vi "getExptComments.vi"(8 "error in (no error)":errorcluster, 11 "Inst.Transport in":refnum<class "Inst.Transport.lvclass">) -> (0 "error out":errorcluster, 2 "comments":string, 3 "Inst.Transport out":refnum<class "Inst.Transport.lvclass">)   [LabVIEW 2019, in "Inst.Transport.lvclass"]
uses:
  Inst.Transport.lvclass
  Typedefs/Inst.Transport.PublicCommands--Enum.ctl
  Typedefs/ExptComments--RequestResponse--Cluster.ctl
  6c876aff-ff84-4813-ac9a-c50593048c18.vi
  6c876aff-ff84-4813-ac9a-c50593048c18.vi/f3aab538-2ba4-4839-a97a-c1727853db43.vi
  6c876aff-ff84-4813-ac9a-c50593048c18.vi/9b28f1f0-4a86-40ce-ac33-3c033e206612.vi
  <vilib>/Utility/Data Type/Get Type Information.vi
  <vilib>/JDP Science/JSONtext/JSON text to Variant.vi
  <vilib>/JDP Science/JSONtext/LVClass Serializer/JSONtext LVClass Serializer.lvclass
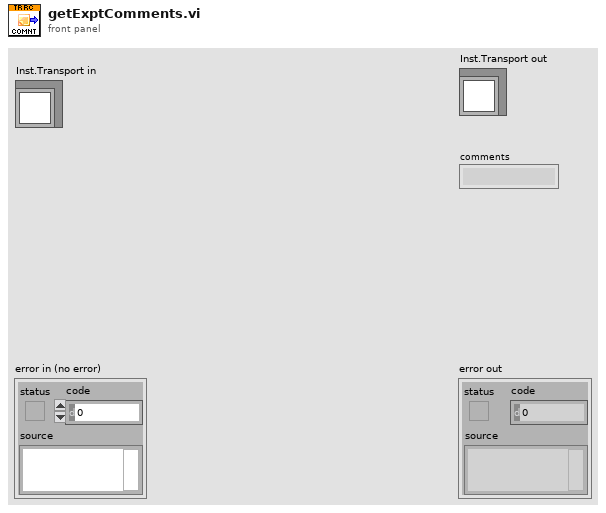
[diagram p1: front panel]
types:
  T1 = typedef "Inst.Transport.lvclass/ExptComments--RequestResponse--Cluster.ctl" = cluster{"comments":string}
  T2 = typedef "Inst.Transport.lvclass/Inst.Transport.PublicCommands--Enum.ctl" = enum16{"startTransport", "stopTransport", "getStatus", "setExptFolder", "getExptFolder", "setExptComments", "getExptComments", "setExptParam", "appendExptParam", "clearExptParam", "setSweepConfig", "getSweepConfig"}
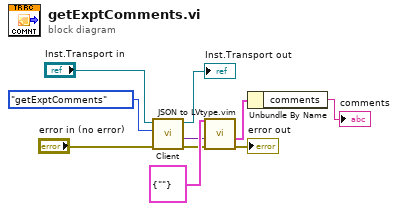
[diagram p0: block diagram]
diagram:
  n1 = call-dynamic "Client.vi"("error in (no error)"="error in (no error)", "Command in"=Inst.Transport.PublicCommands--Enum."getExptComments" ("Commands"), "Instrument in"="Inst.Transport in") -> ("error out"=w4:errorcluster, "Data out"=w5:variant, "Instrument out"=→"Inst.Transport out":refnum<class "Inst.Transport.lvclass">)  [unwired: 5 in, 1 out]
  n2 = call "JSON to LVtype.vim"("type"=T1 {"comments"=""} ("setExptComments"), "error in (no error)"=w4, "JSON Data in"=w5) -> ("error out"=→"error out":errorcluster, "Data out"=w2:T1)  [unwired: 7 in]
  n3 = Unbundle By Name(w2) -> ("comments"=→"comments":string)
